vi "S30c_dll OpenCom.vi"(5 "Echo (RS485 converter)":bool=TRUE, 6 "error in":errorcluster, 7 "Baudrate":enum16{"9600", "115200"}(ring), 8 "Timeout":i16=50, 9 "ComPort-Nr.":i16=1) -> (0 "error out":errorcluster)   [LabVIEW 2014, in "K_S30c_dll.lvlib"]
uses:
  K_S30c_dll.lvlib
  s30c.dll
panel:
  # "Open ComPort\n\nusing s30c.dll\nKeller AG für Druckmesstechnik, 29.5.08 b.v."
  # "For Keller converter\nRS232 or USB to RS485: ON"
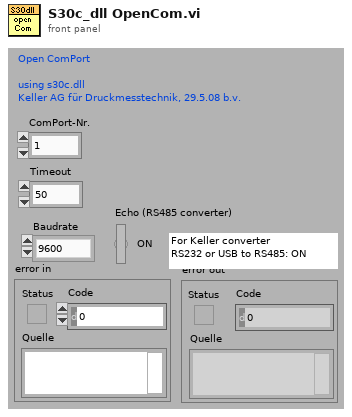
[diagram p1: front panel]
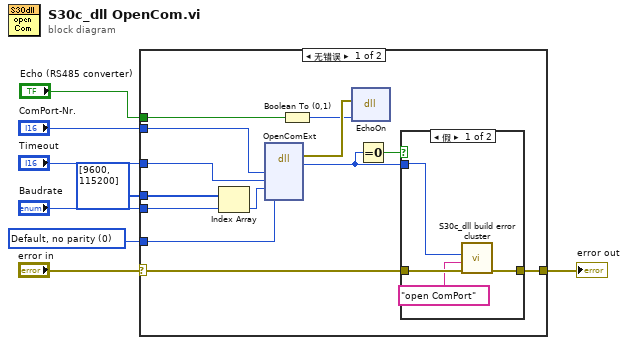
[diagram p0: block diagram]
diagram:
  w1 = i16 0 items=["Default, no parity", "odd parity", "even parity"] ("Parity")
  n1 = case shown="无错误" "error in" {
    selector: "error in" -> [w14 w27]
    tunnel: [w13 w27] -> w3
    tunnel: "ComPort-Nr." -> [w21 _]
    tunnel: "Timeout" -> [w20 _]
    tunnel: w1 -> [w19 _]
    tunnel: "Baudrate" -> [w18 _]
    tunnel: "Echo (RS485 converter)" -> [w10 _]
    tunnel: i32[] [9600, 115200] -> [w9 _]
    frame No Error {
      n2 = Index Array(array=w9, index=w18) -> (element=w17:i32)
      n3 = dll-call lib="PTH2Labs EworkSINOPEC北控自动相渗software2.08.5_dlls30c.dll" fn="OpenComExt"("ComPort"=w21, "Timeout"=w20, "baudrate"=w17, "Parity"=w19) -> (error out=w12:errorcluster, w15:i16)  [unwired: 7 in, 1 out]
      n4 = Boolean To (0,1)(Boolean=w10) -> (0, 1=w11:i16)
      n5 = dll-call lib="PTH2Labs EworkSINOPEC北控自动相渗software2.08.5_dlls30c.dll" fn="EchoOn"(error in=w12, "Echo"=w11) -> ()  [unwired: 4 in, 2 out]
      n6 = Equal To 0?(x=w15) -> (x = 0?=w16:bool)
      n7 = case shown="假" w16 {
        tunnel: w15 -> [w23 _]
        tunnel: w14 -> [w25 w26]
        tunnel: [w24 w26] -> w13
        frame False {
          n8 = call "S30c_dll build error cluster.vi"("error in"=w25, "error Text"="open ComPort", "error code"=w23) -> ("error out"=w24:errorcluster)  [unwired: 4 in]
        }
        frame True {
        }
      }
    }
    frame Error {
    }
  }
  "error out" <- w3
